vi "DTI - Euler Forward.vi"(6 "Init":dbl, 8 "K":dbl=1.0, 9 "Ts":dbl, 10 "U":dbl) -> (2 "Y":dbl)   [LabVIEW 2017]
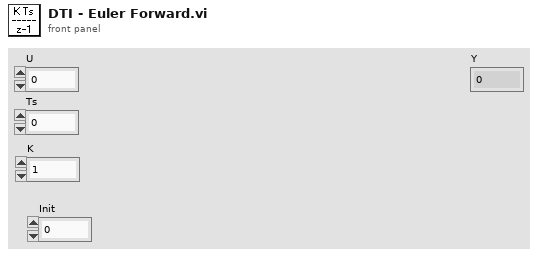
[diagram p1: front panel]
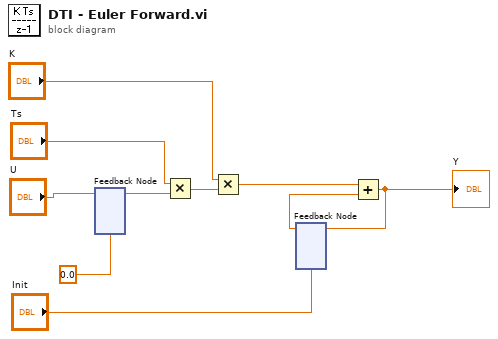
[diagram p0: block diagram]
diagram:
  n1 = feedback #1(0.0) -> (w9:dbl)
  n2 = feedback-in #1("U") -> ()
  n3 = Multiply(x="Ts", y=w9) -> (x*y=w7:dbl)
  n4 = Multiply(x="K", y=w7) -> (x*y=w5:dbl)
  n5 = feedback #2("Init") -> (w4:dbl)
  n6 = Add(x=w5, y=w4) -> (x+y=w3:dbl)
  "Y" <- w3
  n7 = feedback-in #2(w3) -> ()
